vi "Create Oneof Metadata.vi"(8 "error in (no error)":errorcluster, 11 "ProtoFile Oneofs":u64[](array[numeric])) -> (0 "error out":errorcluster, 3 "Oneof Parameters":T1[](array[typedef]))   [LabVIEW 2019, in "gRPC Template Creation Utility.lvlib"]
uses:
  gRPC Template Creation Utility.lvlib
  TypeDefs/Message Element Type.ctl
  TypeDefs/Message Element Metadata (Scripting).ctl
  TypeDefs/Oneof Metadata.ctl
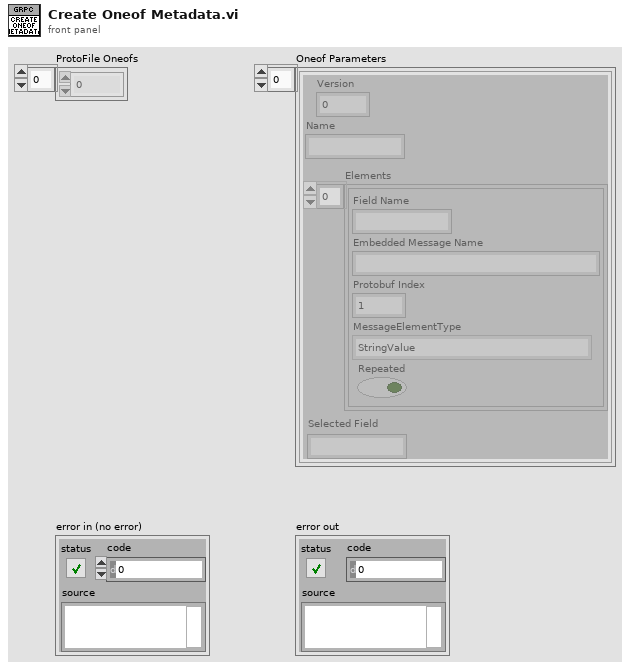
[diagram p1: front panel]
types:
  T1 = typedef "gRPC Template Creation Utility.lvlib/Oneof Metadata.ctl" = cluster{"Version":i32, "Name":string, "Elements":T2[], "Selected Field":string}
  T2 = typedef "gRPC Template Creation Utility.lvlib/Message Element Metadata (Scripting).ctl" = cluster{"Field Name":string, "Embedded Message Name":string, "Protobuf Index":i32, "MessageElementType":T3, "Repeated":bool}
  T3 = typedef "gRPC Template Creation Utility.lvlib/Message Element Type.ctl" = enum32{"Int32Value", "FloatValue", "DoubleValue", "BoolValue", "StringValue", "MessageValue", "Int64Value", "UInt32Value", "UInt64Value", "EnumValue", "Bytes", "Fixed64", "Fixed32", "SFixed64", "SFixed32", "SInt64", "SInt32", "Oneof"}
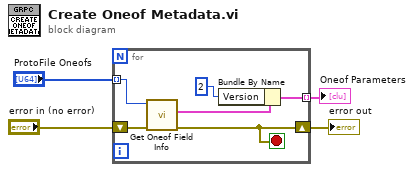
[diagram p0: block diagram]
diagram:
  n1 = for {
    tunnel: "ProtoFile Oneofs" -> [w8] mode=indexing
    shift-right: [w5] -> w4
    shift-left: "error in (no error)" -> [w6]
    tunnel: [w10] -> w1 mode=indexing
    stop <- w5 stop-if-true
    n2 = call "Get Oneof Field Info.vi"("error in (no error)"=w6, "Oneof Field ref in"=w8) -> ("error out"=w5:errorcluster, "Field Info"=w7:T1)  [unwired: 7 in, 1 out]
    n3 = Bundle By Name(cluster=w7, "Version"=2) -> (w10:T1)
  }
  "error out" <- w4
  "Oneof Parameters" <- w1
